vi "LV2GSettings.vi"(7 "Operation":T2=enum."Read File", 8 "error in (no error)":errorcluster, 11 "Settings":T1={"Mono Cr"={"Port"="COM3", "baud rate"=19200, "data bits"=8, "parity"=enum."None", "stop bits"=10, "flow control"=0, "timeout"=2000}, "Merlin"={"Port"="COM4", "baud rate"=9600, "data bits"=8, "parity"=enum."None", "stop bits"=10, "flow control"=0, "timeout"=2000}} {"Merlin"."flow control" items=["None", "XON/XOFF", "RTS/CTS", "XON/XOFF & RTS/CTS", "DTR/DSR", "XON/XOFF & DTR/DSR"]; "Merlin"."stop bits" items=["1.0"=10, "1.5"=15, "2.0"=20]; "Merlin"."data bits" min=5 max=8 step=1; "Mono Cr"."flow control" items=["None", "XON/XOFF", "RTS/CTS", "XON/XOFF & RTS/CTS", "DTR/DSR", "XON/XOFF & DTR/DSR"]; "Mono Cr"."stop bits" items=["1.0"=10, "1.5"=15, "2.0"=20]; "Mono Cr"."data bits" min=5 max=8 step=1}) -> (0 "error out":errorcluster, 3 "Settings out":T1={"Mono Cr"={"Port"="", "baud rate"=9600, "data bits"=8, "parity"=enum."None", "stop bits"=10, "flow control"=0, "timeout"=2000}, "Merlin"={"Port"="", "baud rate"=9600, "data bits"=8, "parity"=enum."None", "stop bits"=10, "flow control"=0, "timeout"=2000}} {"Merlin"."flow control" items=["None", "XON/XOFF", "RTS/CTS", "XON/XOFF & RTS/CTS", "DTR/DSR", "XON/XOFF & DTR/DSR"]; "Merlin"."stop bits" items=["1.0"=10, "1.5"=15, "2.0"=20]; "Merlin"."data bits" min=5 max=8 step=1; "Mono Cr"."flow control" items=["None", "XON/XOFF", "RTS/CTS", "XON/XOFF & RTS/CTS", "DTR/DSR", "XON/XOFF & DTR/DSR"]; "Mono Cr"."stop bits" items=["1.0"=10, "1.5"=15, "2.0"=20]; "Mono Cr"."data bits" min=5 max=8 step=1})   [LabVIEW 2018]
uses:
  Strict Type Controls/Settings Operation.ctl
  Strict Type Controls/Settings.ctl
  <vilib>/Utility/config.llb/Read Key (String).vi
  <vilib>/Utility/config.llb/Write Key (String).vi
  <vilib>/Utility/config.llb/NI_LVConfig.lvlib
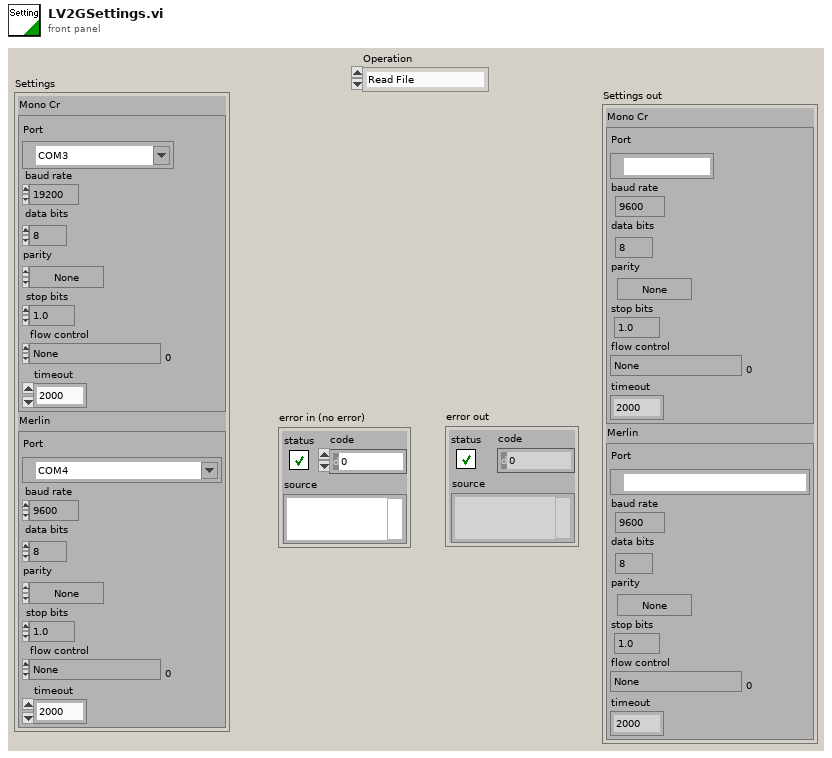
[diagram p1: front panel]
types:
  T1 = typedef "Settings.ctl" = cluster{"Mono Cr":cluster{"Port":refnum<visa-resource-name>, "baud rate":u32, "data bits":u16, "parity":enum16{"None", "Odd", "Even", "Mark", "Space"}, "stop bits":u16, "flow control":u16, "timeout":u32}, "Merlin":cluster{"Port":refnum<visa-resource-name>, "baud rate":u32, "data bits":u16, "parity":enum16{"None", "Odd", "Even", "Mark", "Space"}, "stop bits":u16, "flow control":u16, "timeout":u32}}
  T2 = typedef "Settings Operation.ctl" = enum8{"Get Value", "Set Value", "Read File", "Write File", "Write Stored Value"}
  T3 = typedef "NI_LVConfig.lvlib/Config Data RefNum.ctl" = refnum<k1>
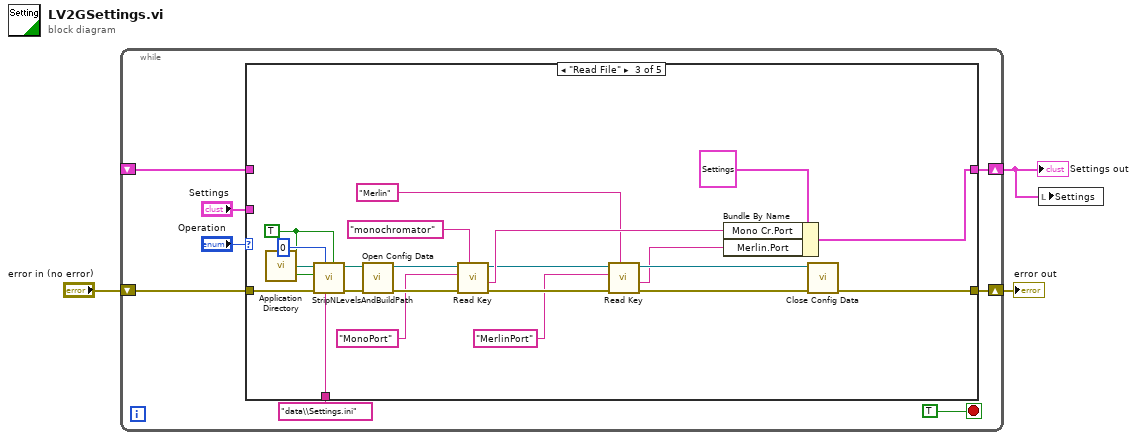
[diagram p0: block diagram]
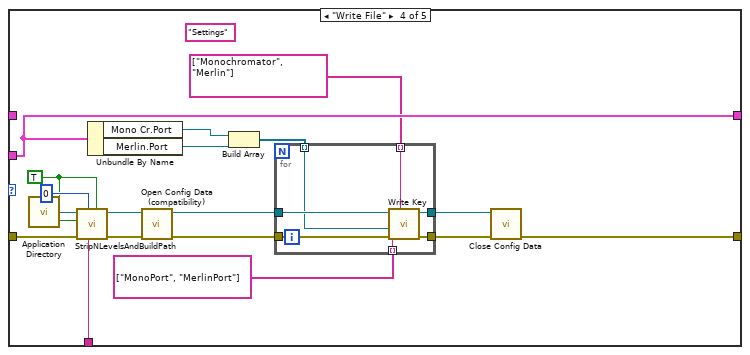
[diagram p4: hidden frame]
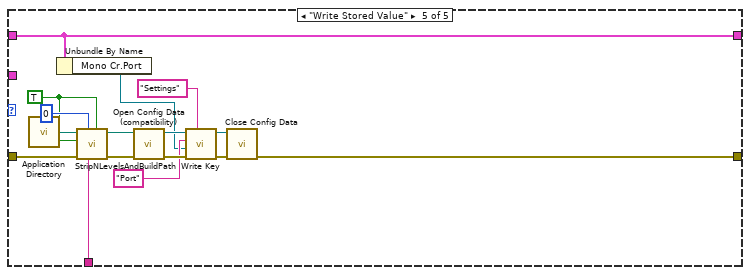
[diagram p5: hidden frame]
diagram:
  n1 = while {
    shift-right: [w10] -> w2
    shift-left: _ -> [w11]
    shift-right: [w7] -> w1
    shift-left: "error in (no error)" -> [w8]
    stop <- TRUE stop-if-true
    n2 = case shown="\"Read File\"" "Operation" {
      tunnel: w11 -> [w13 _ _ _ w66]
      tunnel: [w13 w15 w27 w43 w66] -> w10
      tunnel: "Settings" -> [_ w15 _ w43 _]
      tunnel: w8 -> [w12 w14 w30 w54 w73]
      tunnel: [w12 w14 w25 w45 w72] -> w7
      tunnel: "data\\Settings.ini" ("Build Path") -> [_ _ w29 w44 w71]
      frame "Get Value" {
      }
      frame "Set Value" {
      }
      frame "Read File" {
        w35 = TRUE ("Is File?")
        n3 = call <vilib>:"Application Directory.vi"() -> ("Application Directory"=w37:path)
        n4 = call "StripNLevelsAndBuildPath.vi"("Create Folders"=w35, "Build Path"=w29, "Strip Levels"=0, "error in(no error)"=w30, "Is File"=w35, "Path In"=w37) -> ("error out"=w31:errorcluster, "Path Out"=w34:path)  [unwired: 4 out]
        n5 = call <vilib>:"Open Config Data.vi"("error in (no error)"=w31, "configuration file path"=w34) -> ("error out"=w32:errorcluster, "refnum"=w33:T3)  [unwired: 7 in, 1 out]
        n6 = call-poly <vilib>:"Read Key.vi"("section"="monochromator", "error in (no error)"=w32, "key"="MonoPort", "refnum"=w33) -> ("error out"=w24:errorcluster, "value"=w26:string, "refnum out"=w23:T3)  [unwired: 4 in, 1 out]
        n7 = call-poly <vilib>:"Read Key.vi"("section"="Merlin", "error in (no error)"=w24, "key"="MerlinPort", "refnum"=w23) -> ("error out"=w22:errorcluster, "value"=w20:string, "refnum out"=w21:T3)  [unwired: 4 in, 1 out]
        n8 = Bundle By Name(cluster=T1 {"Mono Cr"={"Port"="", "baud rate"=9600, "data bits"=8, "parity"=enum."None", "stop bits"=10, "flow control"=0, "timeout"=2000}, "Merlin"={"Port"="", "baud rate"=9600, "data bits"=8, "parity"=enum."None", "stop bits"=10, "flow control"=0, "timeout"=2000}} ("Settings"), "Mono Cr.Port"=w26, "Merlin.Port"=w20) -> (w27:T1)
        n9 = call <vilib>:"Close Config Data.vi"("error in (no error)"=w22, "refnum"=w21) -> ("error out"=w25:errorcluster)  [unwired: 1 in, 8 out]
      }
      frame "Write File" {
        (unwired) "Settings" ("section")
        w52 = TRUE ("Is File?")
        n10 = call <vilib>:"Application Directory.vi"() -> ("Application Directory"=w55:path)
        n11 = call "StripNLevelsAndBuildPath.vi"("Create Folders"=w52, "Build Path"=w44, "Strip Levels"=0, "error in(no error)"=w54, "Is File"=w52, "Path In"=w55) -> ("error out"=w46:errorcluster, "Path Out"=w51:path)  [unwired: 4 out]
        n12 = Unbundle By Name(w43) -> ("Mono Cr.Port"=w42:refnum<visa-resource-name>, "Merlin.Port"=w41:refnum<visa-resource-name>)
        n13 = call <vilib>:"Open Config Data (compatibility).vi"("error in (no error)"=w46, "configuration file path"=w51) -> ("error out"=w49:errorcluster, "refnum"=w50:T3)  [unwired: 7 in, 1 out]
        n14 = Build Array(w42, w41) -> (w39:refnum<visa-resource-name>[])
        n15 = for {
          tunnel: string[] ["MonoPort", "MerlinPort"] -> [w58] mode=indexing
          tunnel: w49 -> [w61]
          tunnel: [w60] -> w48
          tunnel: w50 -> [w62]
          tunnel: [w59] -> w47
          tunnel: w39 -> [w57] mode=indexing
          tunnel: string[] ["Monochromator", "Merlin"] -> [w56] mode=indexing
          n16 = call-poly <vilib>:"Write Key.vi"("section"=w56, "error in (no error)"=w61, "value"=w57, "key"=w58, "refnum"=w62) -> ("error out"=w60:errorcluster, "refnum out"=w59:T3)  [unwired: 4 in, 1 out]
        }
        n17 = call <vilib>:"Close Config Data.vi"("error in (no error)"=w48, "refnum"=w47) -> ("error out"=w45:errorcluster)  [unwired: 1 in, 8 out]
      }
      frame "Write Stored Value" {
        w76 = TRUE ("Is File?")
        n18 = call <vilib>:"Application Directory.vi"() -> ("Application Directory"=w78:path)
        n19 = Unbundle By Name(w66) -> ("Mono Cr.Port"=w63:refnum<visa-resource-name>)
        n20 = call "StripNLevelsAndBuildPath.vi"("Create Folders"=w76, "Build Path"=w71, "Strip Levels"=0, "error in(no error)"=w73, "Is File"=w76, "Path In"=w78) -> ("error out"=w74:errorcluster, "Path Out"=w75:path)  [unwired: 4 out]
        n21 = call <vilib>:"Open Config Data (compatibility).vi"("error in (no error)"=w74, "configuration file path"=w75) -> ("error out"=w68:errorcluster, "refnum"=w70:T3)  [unwired: 7 in, 1 out]
        n22 = call-poly <vilib>:"Write Key.vi"("section"="Settings", "error in (no error)"=w68, "value"=w63, "key"="Port", "refnum"=w70) -> ("error out"=w67:errorcluster, "refnum out"=w69:T3)  [unwired: 4 in, 1 out]
        n23 = call <vilib>:"Close Config Data.vi"("error in (no error)"=w67, "refnum"=w69) -> ("error out"=w72:errorcluster)  [unwired: 1 in, 8 out]
      }
    }
  }
  "error out" <- w1
  "Settings out" <- w2
  n24 = local write "Settings"(w2) -> ()
